vi "Day 11 Task 1.vi"() -> ()   [LabVIEW 2018]
panel:
  out "step":i32
  out "State before flash":i32[][](array[numeric])
  out "State Now":i32[][](array[numeric])
  out "Flash":bool[][](array[boolean])
  out "while loop i":i32
  out "State at Start":i32[][](array[numeric])
  in  "Number of steps":i32=11
  out "Number of flashes (part 1)":i32
  out "State at end":i32[][](array[numeric])
  # "Before any steps:\n11111\n19991\n19191\n19991\n11111\n\nAfter step 1:\n34543\n40004\n50005\n40004\n34543\n\nAfter step 2:\n45654\n51115\n61116\n51115\n45654"
  # "After step 1:\n6594254334\n3856965822\n6375667284\n7252447257\n7468496589\n5278635756\n3287952832\n7993992245\n5957959665\n6394862637"
  # "After step 2:\n8807476555\n5089087054\n8597889608\n8485769600\n8700908800\n6600088989\n6800005943\n0000007456\n9000000876\n8700006848"
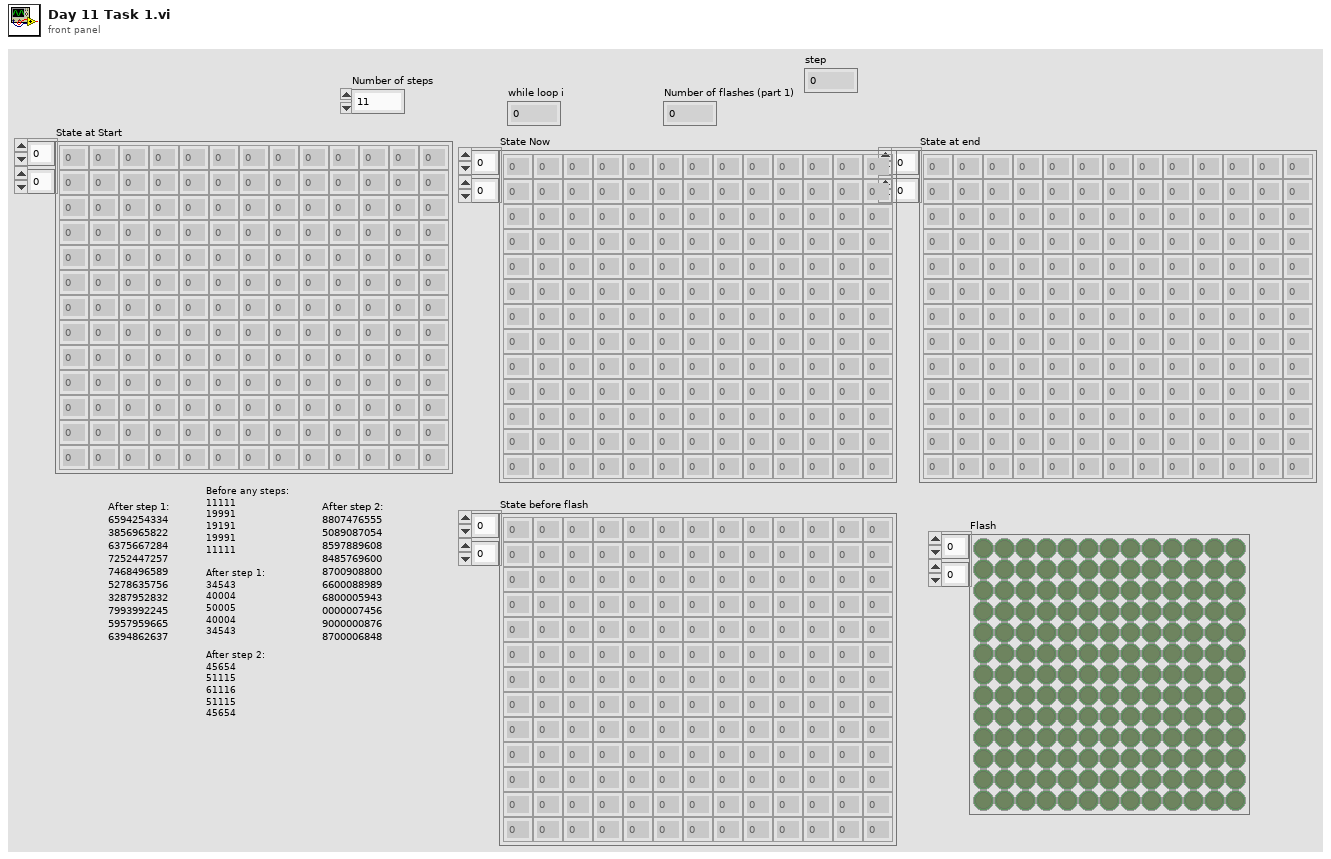
[diagram p1: front panel]
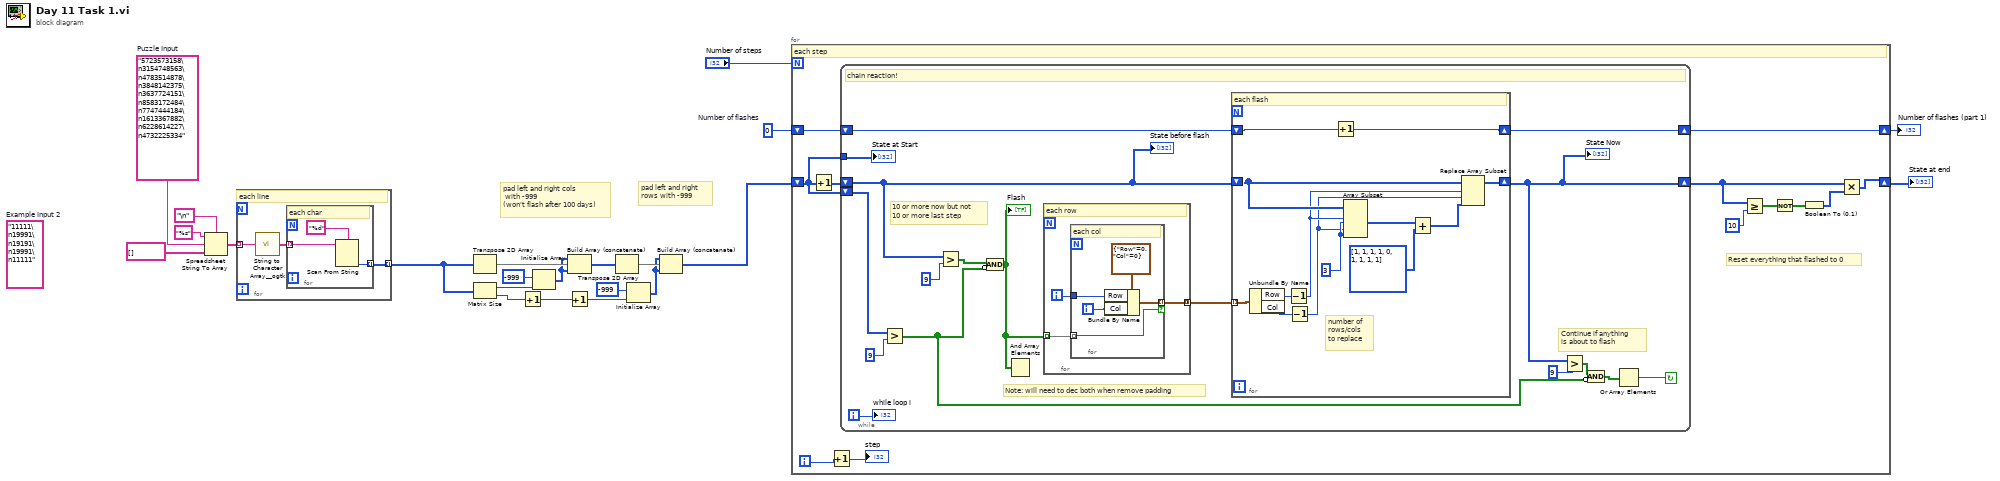
[diagram p0: block diagram]
diagram:
  w1 = "5723573158\n3154748563\n4783514878\n3848142375\n3637724151\n8583172484\n7747444184\n1613367882\n6228614227\n4732225334"  # Puzzle Input
  w4 = 0  # Number of flashes
  (unwired) "11111\n19991\n19191\n19991\n11111"  # Example Input 2
  # "pad left and right \nrows with -999"
  # "pad left and right cols\n with -999 \n(won't flash after 100 days)"
  n1 = Spreadsheet String To Array(delimiter (Tab)="\n", format string="%s", spreadsheet string=w1, array type (2D Dbl)=string[] []) -> (array=w19:string[])
  n2 = for {
    tunnel: w19 -> [w25] mode=indexing
    tunnel: [w23] -> w7 mode=indexing
    # "each line"
    n3 = call <userlib>:"String to Character Array__ogtk.vi"("Input String"=w25) -> ("Character Array"=w24:string[])
    n4 = for {
      tunnel: w24 -> [w28] mode=indexing
      tunnel: [w26] -> w23 mode=indexing
      # "each char"
      n5 = Scan From String(format string="%d", input string=w28) -> (output 1=w26:i32)  [unwired: 3 in, 3 out]
    }
  }
  n6 = Transpose 2D Array(2D array=w7) -> (transposed array=w18:i32[][])
  n7 = Matrix Size(0:w7) -> (1:w14:i32, 2:w11:i32)
  n8 = Increment(x=w11) -> (x+1=w8:i32)
  n9 = Initialize Array(-999 ("element"), w14) -> (w13:i32[])
  n10 = Build Array (concatenate)(w13, w18, w13) -> (w17:i32[][])
  n11 = Increment(x=w8) -> (x+1=w10:i32)
  n12 = Transpose 2D Array(2D array=w17) -> (transposed array=w12:i32[][])
  n13 = Initialize Array(-999 ("number of columns"), w10) -> (w9:i32[])
  n14 = Build Array (concatenate)(w9, w12, w9) -> (w2:i32[][])
  n15 = for {
    N: "Number of steps" -> [_]
    shift-right: [w34] -> w6
    shift-left: w2 -> [w29]
    shift-right: [w39] -> w3
    shift-left: w4 -> [w40]
    i -> [w31]
    # "Reset everything that flashed to 0"
    # "each step"
    n16 = Increment(x=w29) -> (x+1=w32:i32[][])
    n17 = Increment(x=w31) -> (x+1=→"step":i32)
    n18 = while {
      shift-right: [w54] -> w39
      shift-left: w40 -> [w55]
      shift-right: [w44] -> w33
      shift-left: w32 -> [w43]
      shift-left: w29 -> [w42]
      tunnel: w29 -> [w45]
      i -> [w53]
      stop <- w46 continue-if-true
      # "10 or more now but not\n10 or more last step"
      # "Continue if anything \nis about to flash"
      # "Note: will need to dec both when remove padding"
      # "chain reaction!"
      n19 = Greater?(x=w42, y=9) -> (0:w48:bool[][])
      n20 = Greater?(x=w43, y=9) -> (0:w51:bool[][])
      n21 = Compound Arithmetic op=AND(w51, invert w48) -> (w41:bool[][])
      "Flash" <- w41
      n22 = And Array Elements(Boolean array=w41) -> ()  [unwired: 1 out]
      n23 = for {
        tunnel: w41 -> [w73] mode=indexing
        tunnel: [w71] -> w56 mode=concatenating
        i -> [w72]
        # "each row"
        n24 = for {
          tunnel: w73 -> [w76] mode=indexing
          tunnel: w72 -> [w74]
          tunnel: [w77] -> w71 mode=indexing if=w76
          i -> [w75]
          # "each col"
          n25 = Bundle By Name(cluster=cluster{"Row":i32, "Col":i32} {"Row"=0, "Col"=0}, "Row"=w74, "Col"=w75) -> (w77:cluster{"Row":i32, "Col":i32})
        }
      }
      n26 = for {
        tunnel: w56 -> [w70] mode=indexing
        shift-right: [w65] -> w44
        shift-left: w43 -> [w66]
        shift-right: [w64] -> w54
        shift-left: w55 -> [w63]
        w69 = 3 ("length")
        # "number of \nrows/cols\nto replace"
        # "each flash"
        n27 = Unbundle By Name(w70) -> ("Row"=w62:i32, "Col"=w61:i32)
        n28 = Decrement(x=w62) -> (x-1=w60:i32)
        n29 = Decrement(x=w61) -> (x-1=w59:i32)
        n30 = Increment(x=w63) -> (x+1=w64:i32)
        n31 = Array Subset(array=w66, index (row)=w60, length (row)=w69, index (col)=w59, length (col)=w69) -> (w68:i32[][])
        n32 = Add(x=w68, y=i32[][] [[1, 1, 1], [1, 0, 1], [1, 1, 1]]) -> (x+y=w58:i32[][])
        n33 = Replace Array Subset(array=w66, new element=w58, index (row)=w60, index (col)=w59) -> (w65:i32[][])
      }
      "State Now" <- w44
      n34 = Greater?(x=w44, y=9) -> (0:w49:bool[][])
      n35 = Compound Arithmetic op=AND(w49, invert w48) -> (w47:bool[][])
      n36 = Or Array Elements(Boolean array=w47) -> (logical OR=w46:bool)
      "while loop i" <- w53
      "State at Start" <- w45
      "State before flash" <- w43
    }
    n37 = Greater Or Equal?(x=w33, y=10) -> (x >= y?=w37:bool[][])
    n38 = Not(x=w37) -> (.not. x?=w36:bool[][])
    n39 = Boolean To (0,1)(Boolean=w36) -> (0, 1=w35:i16[][])
    n40 = Multiply(x=w33, y=w35) -> (x*y=w34:i32[][])
  }
  "State at end" <- w6
  "Number of flashes (part 1)" <- w3
